vi "Day 1.vi"(8 "Error In":errorcluster) -> (0 "Error Out":errorcluster, 2 "Part 2":u32, 3 "Part 1":u32)   [LabVIEW 2022 SP3]
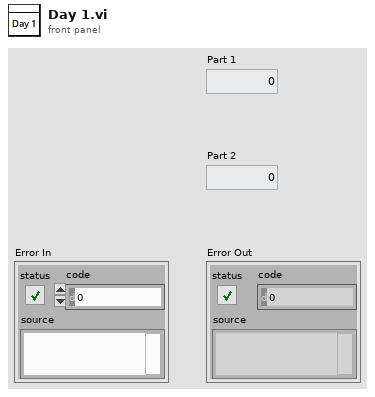
[diagram p1: front panel]
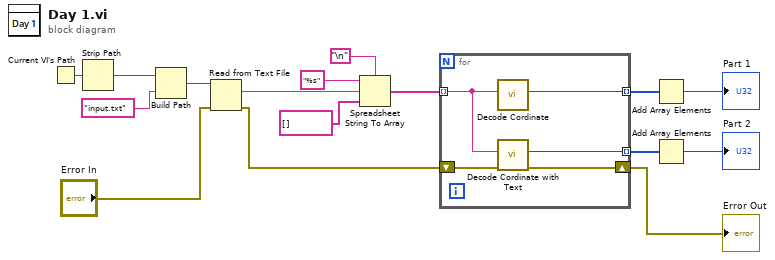
[diagram p0: block diagram]
diagram:
  n1 = Current VI's Path() -> (path=w16:path)
  n2 = Strip Path(path=w16) -> (stripped path=w10:path)  [unwired: 1 out]
  n3 = Build Path(base path=w10, name or relative path="input.txt") -> (appended path=w14:path)
  n4 = Read from Text File(file (use dialog)=w14, error in="Error In") -> (text=w8:string, error out=w2:errorcluster)  [unwired: 2 in, 2 out]
  n5 = Spreadsheet String To Array(delimiter (Tab)="\n", format string="%s" ("spreadsheet string"), spreadsheet string=w8, array type (2D Dbl)=string[] []) -> (array=w7:string[])
  n6 = for {
    tunnel: w7 -> [w20] mode=indexing
    tunnel: [w21] -> w6 mode=indexing
    tunnel: [w19] -> w4 mode=indexing
    shift-right: [w17] -> w1
    shift-left: w2 -> [w18]
    n7 = call "Decode Cordinate.vi"("Encoded Cordinate"=w20) -> ("Decoded Cordinate"=w21:u32)  [unwired: 10 in]
    n8 = call "Decode Cordinate with Text.vi"("Error In"=w18, "Encoded Cordinate"=w20) -> ("Error Out"=w17:errorcluster, "Decoded Cordinate"=w19:u32)  [unwired: 8 in]
  }
  "Error Out" <- w1
  n9 = Add Array Elements(numeric array=w6) -> (sum=→"Part 1":u32)
  n10 = Add Array Elements(numeric array=w4) -> (sum=→"Part 2":u32)
